vi "CreateMark10Monitor.vi"(8 "Error In":errorcluster) -> (0 "Error Out":errorcluster)   [LabVIEW 2019, in "Mark 10 TSTM-DC.lvlib" / "Mark 10 Event Monitor.lvlib"]
uses:
  Mark 10 Event Monitor.lvlib
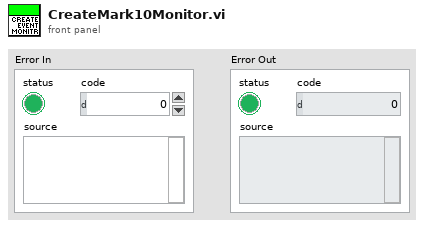
[diagram p1: front panel]
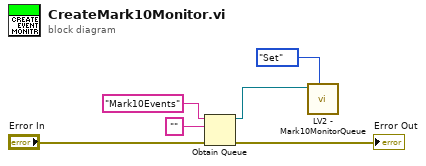
[diagram p0: block diagram]
diagram:
  n1 = Obtain Queue(name (unnamed)="Mark10Events", element data type="", error in (no error)="Error In") -> (queue out=w2:refnum<queue>, error out=→"Error Out":errorcluster)  [unwired: 2 in, 1 out]
  n2 = call "LV2 - Mark10MonitorQueue.vi"("Enum"=enum16{"Set", "Get"}."Set", "Mark10Monitor"=w2) -> ()  [unwired: 9 in, 1 out]
